vi "AddChildtoNode.vi"(8 "error in":errorcluster, 10 "child in":T1, 11 "Engine Parent Editor Node in":refnum<class "Engine Parent Editor Node.lvclass">) -> (0 "error out":errorcluster, 3 "Engine Parent Editor Node out":refnum<class "Engine Parent Editor Node.lvclass">)   [LabVIEW 2013, in "PL Framework Configuration Tool.lvlib" / "Engine Parent Editor Node.lvclass"]
uses:
  Engine Parent Editor Node.lvclass
  Module editor node/module editor node.lvclass
  <vilib>/NI/Module Execution Interface/Engine Configuration/engine configuration.lvclass
  TBM Configuration Node/TBM Configuration Node.lvclass
  <vilib>/NI/CEF/CEF_TreeControl/serializable configuration/NISE_CEF_serializable configuration.lvclass
  <vilib>/NI/CEF/CEF_TreeControl/Node/NISE_CEF_Node.lvclass
  <vilib>/NI/CEF/CEF_TreeControl/Node/NodeRef.ctl
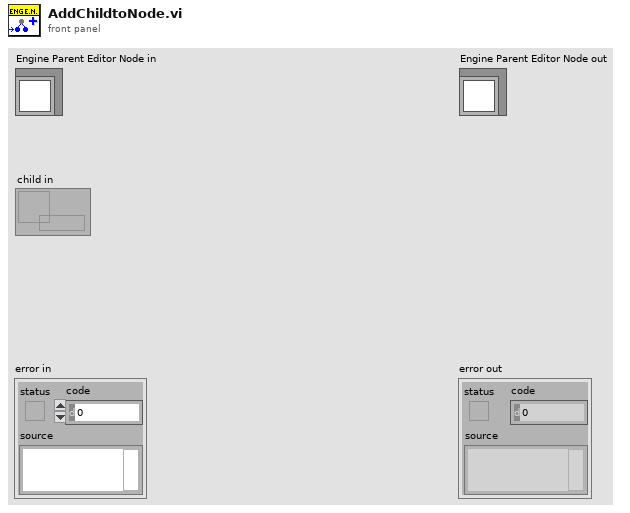
[diagram p1: front panel]
types:
  T1 = typedef "NISE_CEF_Node.lvclass/NodeRef.ctl" = refnum<data-value>
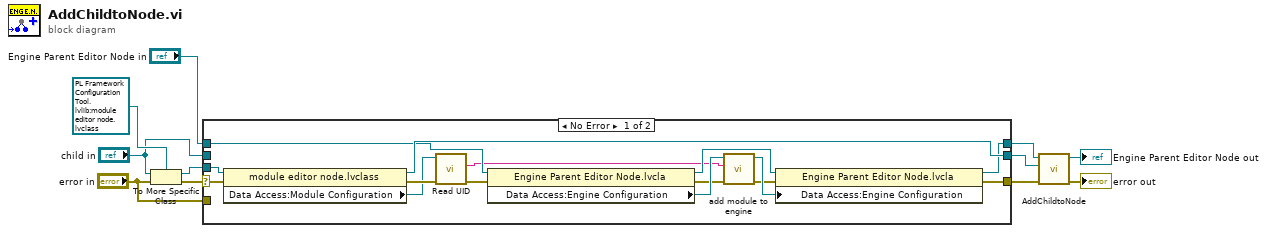
[diagram p0: block diagram]
diagram:
  n1 = To More Specific Class(target class=refnum<data-value> refnum, reference="child in", error in="error in") -> (specific class reference=w8:refnum<data-value>, error out=w6:errorcluster)
  n2 = case shown="No Error" w6 {
    selector: w6 -> [w23 _]
    tunnel: [w17 w29] -> w5
    tunnel: [w25 w28] -> w9
    tunnel: w8 -> [w24 _]
    tunnel: "error in" -> [_ w29]
    tunnel: "child in" -> [_ w28]
    tunnel: "Engine Parent Editor Node in" -> [w21 w27]
    tunnel: [w19 w27] -> w1
    frame No Error {
      n3 = property class="module editor node.lvclass"(reference=w24, error in=w23) -> (reference out=w25:refnum<data-value>, error out=w26:errorcluster, "Data Access:Module Configuration"=w22:refnum<class "TBM module configuration.lvclass">)
      n4 = call <vilib>:"Read UID.vi"("error in"=w26, "configuration in"=w22) -> ("error out"=w20:errorcluster, "instance id"=w12:string)  [unwired: 7 in, 1 out]
      n5 = property class="Engine Parent Editor Node.lvcla"(reference=w21, error in=w20) -> (reference out=w18:refnum<class "Engine Parent Editor Node.lvclass">, error out=w13:errorcluster, "Data Access:Engine Configuration"=w16:refnum<class "engine configuration.lvclass">)
      n6 = call-dynamic "add module to engine.vi"("error in"=w13, "module ID"=w12, "engine configuration in"=w16) -> ("error out"=w14:errorcluster, "engine configuration out"=w15:refnum<class "engine configuration.lvclass">)  [unwired: 7 in]
      n7 = property class="Engine Parent Editor Node.lvcla"(reference=w18, error in=w14, "Data Access:Engine Configuration"=w15) -> (reference out=w19:refnum<class "Engine Parent Editor Node.lvclass">, error out=w17:errorcluster)
    }
    frame Error {
    }
  }
  n8 = call-parent "AddChildtoNode.vi"("error in"=w5, "child in"=w9, "NISE_CEF_Node in"=w1) -> ("error out"=→"error out":errorcluster, "NISE_CEF_Node out"=→"Engine Parent Editor Node out":refnum<class "Engine Parent Editor Node.lvclass">)  [unwired: 7 in]
